vi "Elevator Config.vi"(9 "Elevator Bottom":T1, 11 "Elevator Top":T1) -> ()   [LabVIEW 2012]
uses:
  <vilib>/Rock Robotics/SystemInterfaces/DIO/FPGA_DIOPWMChannel.ctl
  <vilib>/Rock Robotics/WPI/MotorControl/WPI_MotorControlOpen Talon.vi
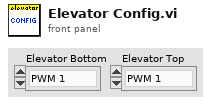
[diagram p1: front panel]
types:
  T1 = typedef "FPGA_DIOPWMChannel.ctl" = enum8{"PWM 1", "PWM 2", "PWM 3", "PWM 4", "PWM 5", "PWM 6", "PWM 7", "PWM 8", "PWM 9", "PWM 10", "Invalid"}
  T2 = typedef "WPI_MotorControlDeviceRef.ctl" = cluster{"DeviceStatus":errorcluster, "Type":enum16{"PWM", "CAN"}, "PWM":cluster{"Digital Module":T3, "PWM Channel":T1, "DeadBand":T4}, "CAN":cluster{"Device Number":u8, "Control Mode":T5, "Semaphore":T6, "Max Vout":dbl}, "Invert":bool, "TransformRef":T7, "InvTransformRef":T7}
  T3 = typedef "FPGA_TypedefDigitalModule.ctl" = enum16{"Digital Module 1", "Digital Module 2"}
  T4 = typedef "WPI_PWMDeadband.ctl" = cluster{"Name":string, "maxPositivePwm":i32, "minPositivePwm":i32, "centerPwm":i32, "maxNegativePwm":i32, "minNegativePwm":i32, "angularRange":u16}
  T5 = typedef "WPI_CANJaguar_ControlMode.ctl" = enum8{"Percent VBus", "Current", "Speed", "Position", "Voltage"}
  T6 = typedef "Semaphore RefNum" = refnum<k1>
  T7 = typedef "WPI_PWMTransform_ConPane.ctl" = refnum<vi>
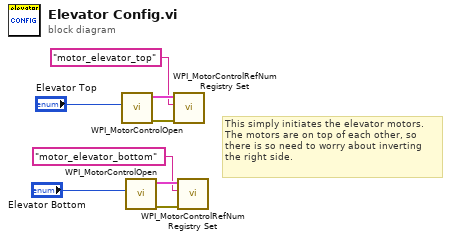
[diagram p0: block diagram]
diagram:
  # "This simply initiates the elevator motors. \nThe motors are on top of each other, so \nthere is so need to worry about inverting\nthe right side."
  n1 = call-poly <vilib>:"WPI_MotorControlOpen.vi"("PWM Channel"="Elevator Top") -> ("error out"=w7:errorcluster, "MotorControlDeviceRef"=w8:T2)  [unwired: 9 in]
  n2 = call-poly <vilib>:"WPI_MotorControlOpen.vi"("PWM Channel"="Elevator Bottom") -> ("error out"=w5:errorcluster, "MotorControlDeviceRef"=w6:T2)  [unwired: 9 in]
  n3 = call <vilib>:"WPI_MotorControlRefNum Registry Set.vi"("error in (no error)"=w7, "refnum name"="motor_elevator_top", "MotorControlDevRef"=w8) -> ()  [unwired: 7 in, 2 out]
  n4 = call <vilib>:"WPI_MotorControlRefNum Registry Set.vi"("error in (no error)"=w5, "refnum name"="motor_elevator_bottom", "MotorControlDevRef"=w6) -> ()  [unwired: 7 in, 2 out]
